vi "Find Store Type.vi"(8 "Message":refnum<class "TestManagerMsg.lvclass">, 11 "Test Event Storage in":refnum<class "Test Event Storage.lvclass">) -> (0 "Message dup":refnum<class "TestManagerMsg.lvclass">, 1 "Store Message":bool, 2 "Store Type":T1, 3 "Test Event Storage out":refnum<class "Test Event Storage.lvclass">)   [LabVIEW 2013, in "Caraya.lvlib" / "Test Event Storage.lvclass"]
uses:
  Test Event Storage.lvclass
  Store Type -- enum.ctl
  Test Manager Message/TestManagerMsg.lvclass
  Test Manager Message Assertion/TestManagerMsg.Assertion.lvclass
  Test Manager Message/TestManagerMsg.lvclass/TestManagerMsg.ctl
  Test Event Storage.lvclass/Test Event Storage.ctl
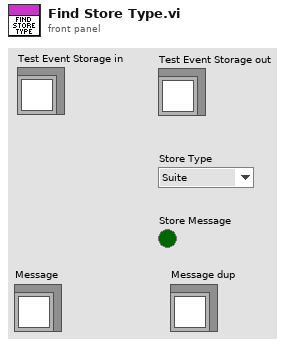
[diagram p1: front panel]
types:
  T1 = typedef "Caraya.lvlib/Test Event Storage.lvclass/Store Type -- enum.ctl" = enum16{"Suite", "Test", "Assert", "none"}
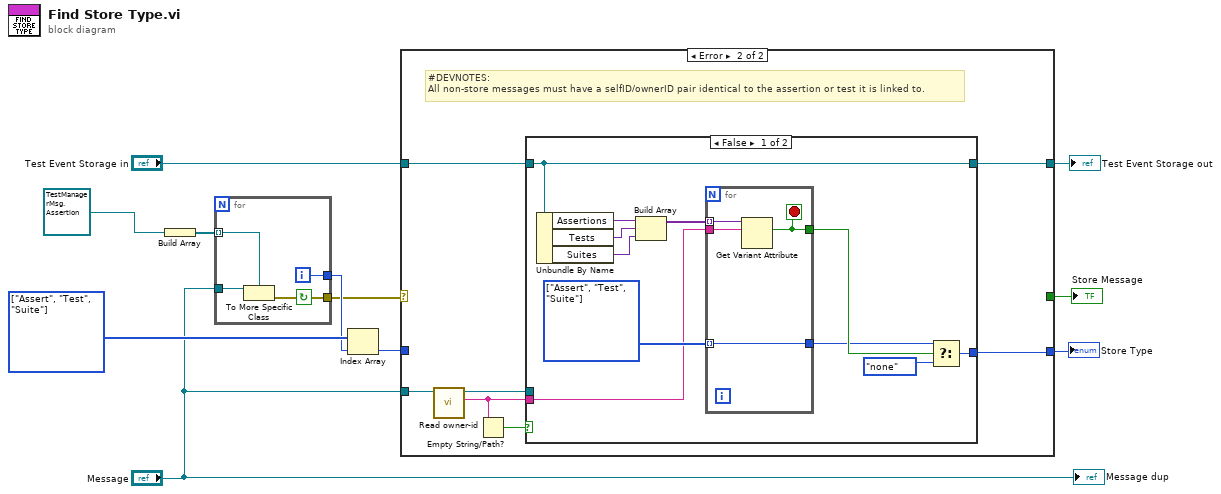
[diagram p0: block diagram]
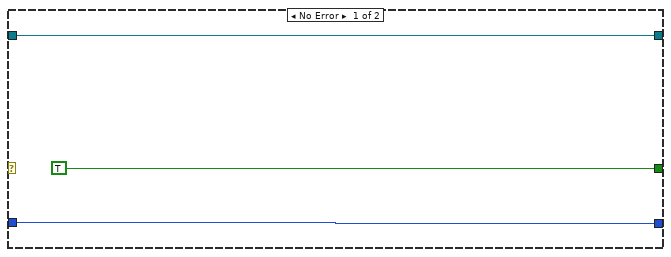
[diagram p2: hidden frame]
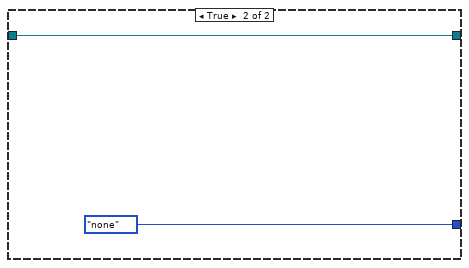
[diagram p3: hidden frame]
diagram:
  w7 = T1[] [enum."Assert", enum."Test", enum."Suite"] items=["Suite", "Test", "Assert", "none"]
  n1 = Build Array(refnum<class "TestManagerMsg.Assertion.lvclass"> refnum ("Caraya.lvlib:TestManagerMsg.Assertion.lvclass")) -> (w8:refnum<class "TestManagerMsg.Assertion.lvclass">[])
  n2 = for {
    tunnel: w8 -> [w14] mode=indexing
    tunnel: "Message" -> [w15]
    tunnel: [w13] -> w6
    tunnel: [w12] -> w4
    i -> [w13]
    stop <- w12 continue-if-true
    n3 = To More Specific Class(target class=w14, reference=w15) -> (error out=w12:errorcluster)  [unwired: 1 in, 1 out]
  }
  n4 = Index Array(array=w7, index=w6) -> (element=w5:T1)
  n5 = case shown="Error" w4 {
    tunnel: "Test Event Storage in" -> [w17 w25]
    tunnel: [w18 w23] -> w10
    tunnel: [w17 w24] -> w9
    tunnel: "Message" -> [_ w21]
    tunnel: w5 -> [w18 _]
    tunnel: [TRUE _] -> w2
    frame No Error {
    }
    frame Error {
      # "#DEVNOTES: \nAll non-store messages must have a selfID/ownerID pair identical to the assertion or test it is linked to."
      n6 = call "Read owner-id.vi"("TestManagerMsg in"=w21) -> ("owner-id"=w19:string, "TestManagerMsg out"=w20:refnum<class "TestManagerMsg.lvclass">)  [unwired: 9 in]
      n7 = Empty String/Path?(string/path=w19) -> (empty?=w22:bool)
      n8 = case shown="False" w22 {
        tunnel: w25 -> [w34 w42]
        tunnel: [w35 Store_Type_--_enum."none" ("Store Type")] -> w23
        tunnel: w19 -> [w26 _]
        tunnel: w20 -> [_ _]
        tunnel: [w34 w42] -> w24
        frame False {
          w28 = T1[] [enum."Assert", enum."Test", enum."Suite"] items=["Suite", "Test", "Assert", "none"]
          n9 = Unbundle By Name(w34) -> ("Assertions"=w31:variant, "Tests"=w32:variant, "Suites"=w29:variant)
          n10 = Build Array(w31, w32, w29) -> (w30:variant[])
          n11 = for {
            tunnel: [w38] -> w33
            tunnel: w26 -> [w40]
            tunnel: w30 -> [w39] mode=indexing
            tunnel: w28 -> [w37] mode=indexing
            tunnel: [w37] -> w27
            stop <- w38 stop-if-true
            n12 = Get Variant Attribute(Variant=w39, name=w40) -> (found=w38:bool)  [unwired: 2 in, 3 out]
          }
          n13 = Select(t=w27, s=w33, f=Store_Type_--_enum."none" ("Store Type")) -> (s? t:f=w35:T1)
        }
        frame True {
        }
      }
    }
  }
  "Store Type" <- w10
  "Test Event Storage out" <- w9
  "Store Message" <- w2
  "Message dup" <- "Message"
